vi "ActionVIOnCompile.vi"(8 "error in (no error)":errorcluster, 11 "Device Item Ref in":T1 format="%.0x") -> (0 "error out":errorcluster)   [LabVIEW 2019, in "TimingDRV System Explorer.lvlib"]
uses:
  TimingDRV System Explorer.lvlib
  <vilib>/NI VeriStand/Custom Device API/Custom Device Item Ref.ctl
  <vilib>/NI VeriStand/Custom Device API/Custom Device API.lvlib
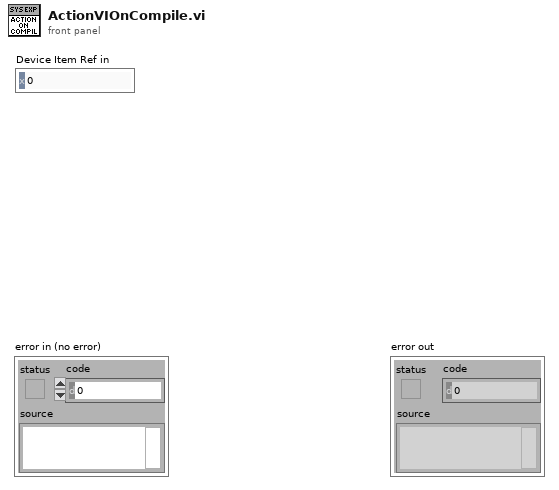
[diagram p1: front panel]
types:
  T1 = typedef "Custom Device API.lvlib/Custom Device Item Ref.ctl" = u64
  T2 = typedef "TimingDRV System Explorer.lvlib/Operating Mode Types.ctl" = enum16{"Free Running", "Single Stepping"}
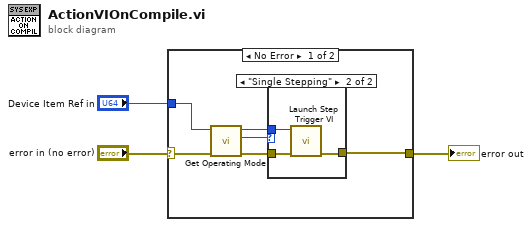
[diagram p0: block diagram]
diagram:
  n1 = case shown="No Error" "error in (no error)" {
    selector: "error in (no error)" -> [w9 w14]
    tunnel: [w6 w14] -> w2
    tunnel: "Device Item Ref in" -> [w5 _]
    frame No Error {
      n2 = call "Get Operating Mode.vi"("error in (no error)"=w9, "Item Ref in"=w5) -> ("error out"=w8:errorcluster, "Operating mode"=w7:T2, "Item Ref out"=w4:T1)  [unwired: 7 in]
      n3 = case shown="\"Single Stepping\"" w7 {
        tunnel: w8 -> [w10 w13]
        tunnel: [w10 w12] -> w6
        tunnel: w4 -> [_ w11]
        frame "Free Running", Default {
        }
        frame "Single Stepping" {
          n4 = call "Launch Step Trigger VI.vi"("error in (no error)"=w13, "Device Item Ref in"=w11) -> ("error out"=w12:errorcluster)  [unwired: 9 in]
        }
      }
    }
    frame Error {
    }
  }
  "error out" <- w2
